vi "Server Connection Callback.vi"(7 "Owner":refnum<class>, 8 "error in (no error)":errorcluster, 9 "Context":variant, 10 "Connection State":T1, 11 "Connection":refnum<class "Connection.lvclass">) -> (0 "error out":errorcluster)   [LabVIEW 2024, in "Stream-TCP.lvlib" / "TCP Server.lvclass"]
uses:
  TCP Server.lvclass
  lv-stream/stream/Connection/Connection.lvclass
  lv-stream/stream/Connection State.ctl
  TCP Client/TCP Client.lvclass
  TCP Server.lvclass/TCP Server.ctl
  lv-stream/stream/Stream.lvlib
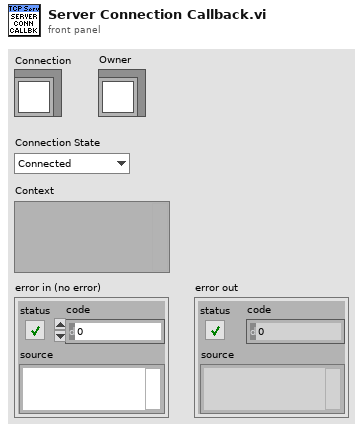
[diagram p1: front panel]
types:
  T1 = typedef "Stream.lvlib/Connection State.ctl" = enum16{"Connected", "Disconnected"}
  T2 = typedef "Stream-TCP.lvlib/TCP Server.lvclass/Ref Data.ctl" = cluster{"Listener":refnum<k5>, "Clients":refnum<class "TCP Client.lvclass">[], "Server Loop":bool}
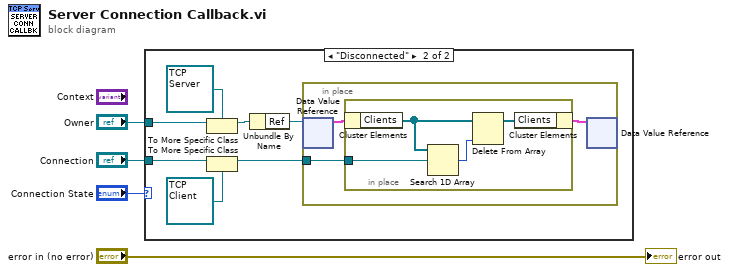
[diagram p0: block diagram]
diagram:
  n1 = case shown="\"Disconnected\"" "Connection State" {
    tunnel: "Owner" -> [_ w11]
    tunnel: "Connection" -> [_ w7]
    frame "Connected" {
    }
    frame "Disconnected" {
      n2 = To More Specific Class(target class=refnum<class "TCP Server.lvclass"> refnum ("Stream-TCP.lvlib:TCP Server.lvclass"), reference=w11) -> (specific class reference=w8:refnum<class "TCP Server.lvclass">)  [unwired: 1 in, 1 out]
      n3 = To More Specific Class(target class=refnum<class "TCP Client.lvclass"> refnum ("Stream-TCP.lvlib:TCP Client.lvclass"), reference=w7) -> (specific class reference=w6:refnum<class "TCP Client.lvclass">)  [unwired: 1 in, 1 out]
      n4 = Unbundle By Name(w8) -> ("Ref"=w9:refnum<data-value>)
      n5 = in-place {
        in-place-border: w6 -> [w12]
        n6 = in-place-dvr #1(w9) -> (w14:T2)  [unwired: 1 out]
        n7 = in-place {
          in-place-border: w12 -> [w18]
          n8 = in-place-cluster #2(w14) -> ("Clients"=w17:refnum<class "TCP Client.lvclass">[])
          n9 = Search 1D Array(1D array=w17, element=w18) -> (index of element=w15:i32)  [unwired: 1 in]
          n10 = Delete From Array(array=w17, index=w15) -> (array with subset deleted=w16:refnum<class "TCP Client.lvclass">[])  [unwired: 1 in, 1 out]
          n11 = in-place-cluster #2("Clients"=w16) -> (w13:T2)
        }
        n12 = in-place-dvr #1(w13) -> ()  [unwired: 2 out]
      }
    }
  }
  "error out" <- "error in (no error)"
